vi "Cleanup Session.vi"(8 "error in (no error)":errorcluster, 11 "RandomNumberGenerator in":refnum<class "RandomNumberGenerator.lvclass">) -> (0 "error out":errorcluster, 3 "RandomNumberGenerator out":refnum<class "RandomNumberGenerator.lvclass">)   [LabVIEW 2020, in "RandomNumberGenerator.lvlib" / "RandomNumberGenerator.lvclass"]
doc: "<b>Cleanup Session</b>\nThis method is used to close any references opened in Configure Session and flush any buffers used.\n\nThis method is followed by either Configure Session (if the plugin is restarting) or Finalize (if the plugin is shutting down)."
uses:
  RandomNumberGenerator.lvclass
  RandomNumberGenerator.lvclass/RandomNumberGenerator.ctl
  <vilib>/ADAS Record/Utilities/ADAS Utilities.lvlib
  C:/Program Files/National Instruments/LabVIEW 2020/vi.lib/FlexLogger/SDK/PluginSDK.lvlibp/PEFClasses/SDK/Processing Element/Processing Element.lvclass
  C:/Projects/GitHub/data-record-ad/IO Plugins/RandomNumberGenerator/PE/RandomNumberGenerator.lvclass
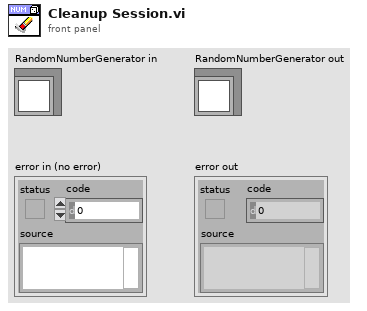
[diagram p1: front panel]
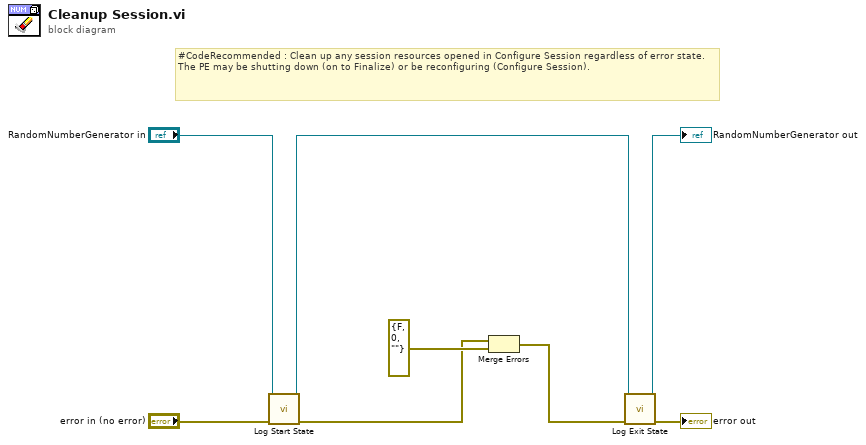
[diagram p0: block diagram]
diagram:
  # "#CodeRecommended : Clean up any session resources opened in Configure Session regardless of error state. The PE may be shutting down (on to Finalize) or be reconfiguring (Configure Session)."
  n1 = call <vilib>:"Log Start State.vi"("error in (no error)"="error in (no error)", "PluginSDK.lvlibp:Processing Element.lvclass"="RandomNumberGenerator in") -> ("error out"=w6:errorcluster, "PluginSDK.lvlibp:Processing Element.lvclass"=w2:refnum<class "RandomNumberGenerator.lvclass">)  [unwired: 8 in]
  n2 = Merge Errors(w6, errorcluster {"status"=FALSE, "code"=0, "source"=""} ("error in")) -> (w4:errorcluster)
  n3 = call <vilib>:"Log Exit State.vi"("error in (no error)"=w4, "PluginSDK.lvlibp:Processing Element.lvclass"=w2) -> ("error out"=→"error out":errorcluster, "PluginSDK.lvlibp:Processing Element.lvclass"=→"RandomNumberGenerator out":refnum<class "RandomNumberGenerator.lvclass">)  [unwired: 8 in]
